vi "JiLTestBAD.vi"() -> ()   [LabVIEW 2015]
panel:
  out "time":dbl
  in  "doublein":dbl(slide) scale=-100.0..100.0
  out "doubleout":dbl
  in  "stringin":string="hola"
  in  "booleanin":bool
  out "booleanout":bool
  out "stringout":string="hola"
  in  "stop":bool
  out "intout":i32
  in  "intin":i32
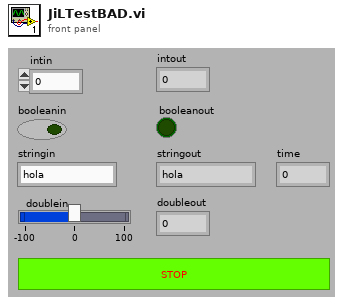
[diagram p1: front panel]
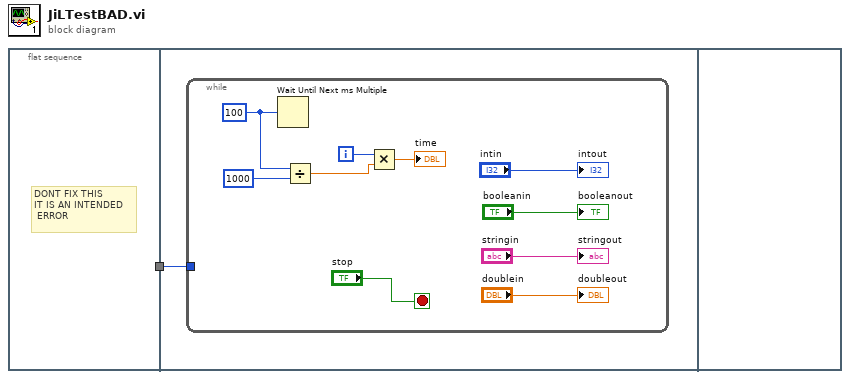
[diagram p0: block diagram]
diagram:
  n1 = flat-sequence {
    tunnel: [w2] -> w1
    tunnel: w1 -> [w3]
    frame #0 {
      # "DONT FIX THIS\nIT IS AN INTENDED\n ERROR"
    }
    frame #1 {
      n2 = while {
        tunnel: [_] -> w3
        i -> [w9]
        stop <- "stop" stop-if-true
        w10 = u32 100 ("millisecond multiple")
        n3 = Wait Until Next ms Multiple(millisecond multiple=w10) -> ()  [unwired: 1 out]
        n4 = Divide(x=w10, y=i64 1000) -> (x/y=w12:dbl)
        n5 = Multiply(x=w9, y=w12) -> (x*y=→"time":dbl)
        "intout" <- "intin"
        "stringout" <- "stringin"
        "booleanout" <- "booleanin"
        "doubleout" <- "doublein"
      }
    }
    frame #2 {
    }
  }
